vi "GetEventForceActuatorWarningField.vi"(10 "Event Data":string, 11 "Cluster in":refnum<vi>) -> (3 "Array":string[](array[string]))   [LabVIEW 2016]
uses:
  SALLV_m1m3/DataTypes/logevent_ForceActuatorWarning.ctl
  SALLV_m1m3/SALLV_m1m3.lvlib
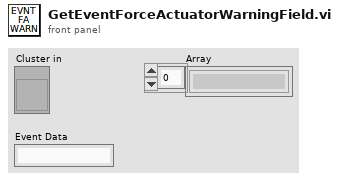
[diagram p1: front panel]
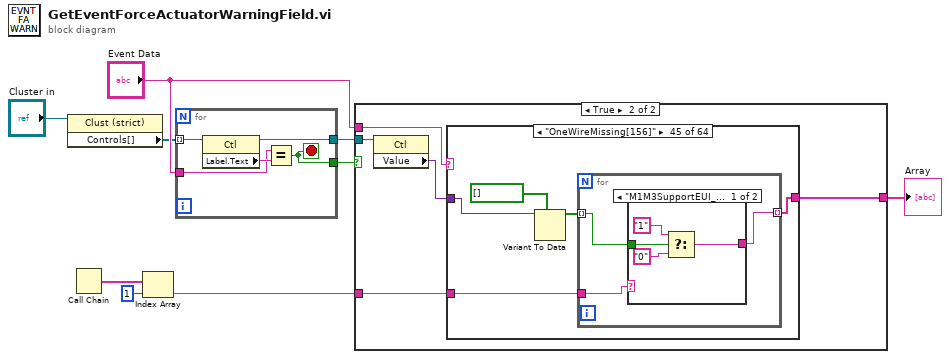
[diagram p0: block diagram]
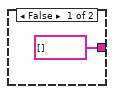
[diagram p2: hidden frame]
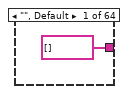
[diagram p3: hidden frame]
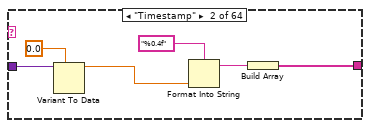
[diagram p4: hidden frame]
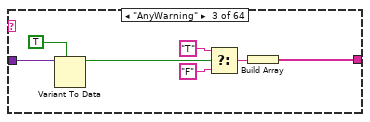
[diagram p5: hidden frame]
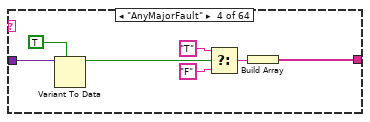
[diagram p6: hidden frame]
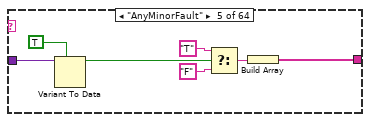
[diagram p7: hidden frame]
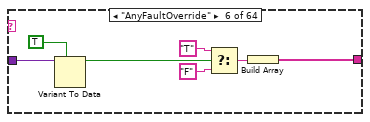
[diagram p8: hidden frame]
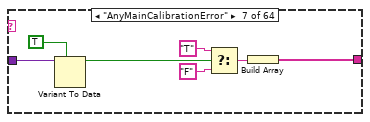
[diagram p9: hidden frame]
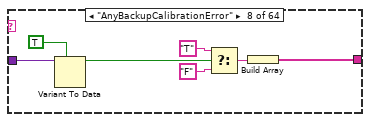
[diagram p10: hidden frame]
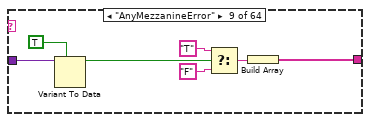
[diagram p11: hidden frame]
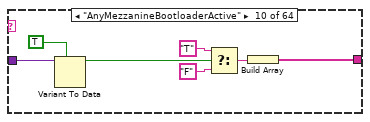
[diagram p12: hidden frame]
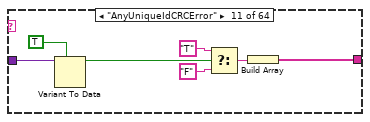
[diagram p13: hidden frame]
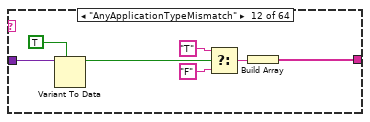
[diagram p14: hidden frame]
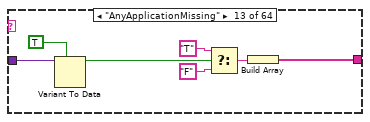
[diagram p15: hidden frame]
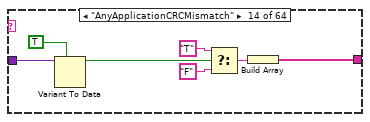
[diagram p16: hidden frame]
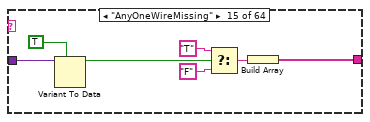
[diagram p17: hidden frame]
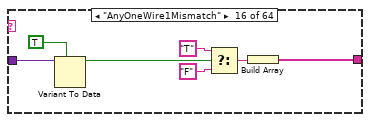
[diagram p18: hidden frame]
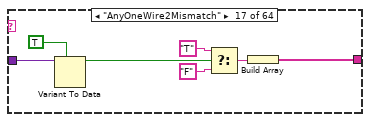
[diagram p19: hidden frame]
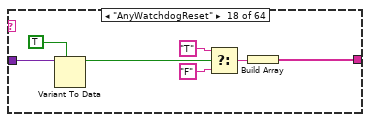
[diagram p20: hidden frame]
diagram:
  n1 = property on="Property Node" class="Clust (strict)"(reference="Cluster in") -> ("Controls[]"=w6:refnum<vi>[])  [unwired: 1 in, 2 out]
  n2 = Call Chain() -> (call chain=w2:string[])
  n3 = Index Array(array=w2, index=1) -> (element=w1:string)
  n4 = for {
    tunnel: w6 -> [w14] mode=indexing
    tunnel: [w13] -> w8
    tunnel: "Event Data" -> [w11]
    tunnel: [w10] -> w9
    stop <- w10 stop-if-true
    n5 = property on="Property Node" class="Ctl"(reference=w14) -> (reference out=w13:refnum<vi>, "Label.Text"=w12:string)  [unwired: 1 in, 1 out]
    n6 = Equal?(x=w11, y=w12) -> (x = y?=w10:bool)
  }
  n7 = case shown="True" w9 {
    tunnel: "Event Data" -> [_ w20]
    tunnel: w8 -> [_ w19]
    tunnel: [string[] [] w17] -> w5
    tunnel: w1 -> [_ w16]
    frame False {
    }
    frame True {
      n8 = property on="Property Node" class="Ctl"(reference=w19) -> ("Value"=w18:variant)  [unwired: 1 in, 2 out]
      n9 = case shown="\"OneWireMissing[156]\"" w20 {
        tunnel: [string[] [] w25 w28 w35 w42 w49 w56 w63 w70 w77 w84 w91 w98 w105 w112 w119 w126 w133 w140 w147 w154 w161 w168 w175 w182 w189 w196 w203 w210 w217 w224 w231 w238 w246 w262 w278 w294 w310 w326 w342 w358 w374 w390 w406 w422 w438 w454 w470 w486 w502 w518 w534 w550 w566 w582 w598 w614 w630 w646 w662 w678 w694 w710 w728] -> w17
        tunnel: w18 -> [_ w23 w34 w41 w48 w55 w62 w69 w76 w83 w90 w97 w104 w111 w118 w125 w132 w139 w146 w153 w160 w167 w174 w181 w188 w195 w202 w209 w216 w223 w230 w237 w244 w249 w265 w281 w297 w313 w329 w345 w361 w377 w393 w409 w425 w441 w457 w473 w489 w505 w521 w537 w553 w569 w585 w601 w617 w633 w649 w665 w681 w697 w713 w726]
        tunnel: w16 -> [_ _ _ _ _ _ _ _ _ _ _ _ _ _ _ _ _ _ _ _ _ _ _ _ _ _ _ _ _ _ _ _ _ w245 w261 w277 w293 w309 w325 w341 w357 w373 w389 w405 w421 w437 w453 w469 w485 w501 w517 w533 w549 w565 w581 w597 w613 w629 w645 w661 w677 w693 w709 _]
        frame "", Default {
        }
        frame "Timestamp" {
          n10 = Variant To Data(type=0.0, Variant=w23) -> (data=w24:dbl)  [unwired: 1 in, 1 out]
          n11 = Format Into String(format string="%0.4f", w24) -> (resulting string=w26:string)  [unwired: 2 in, 1 out]
          n12 = Build Array(w26) -> (w25:string[])
        }
        frame "AnyWarning" {
          n13 = Variant To Data(type=TRUE, Variant=w34) -> (data=w32:bool)  [unwired: 1 in, 1 out]
          n14 = Select(t="T", s=w32, f="F") -> (s? t:f=w29:string)
          n15 = Build Array(w29) -> (w28:string[])
        }
        frame "AnyMajorFault" {
          n16 = Variant To Data(type=TRUE, Variant=w41) -> (data=w39:bool)  [unwired: 1 in, 1 out]
          n17 = Select(t="T", s=w39, f="F") -> (s? t:f=w36:string)
          n18 = Build Array(w36) -> (w35:string[])
        }
        frame "AnyMinorFault" {
          n19 = Variant To Data(type=TRUE, Variant=w48) -> (data=w46:bool)  [unwired: 1 in, 1 out]
          n20 = Select(t="T", s=w46, f="F") -> (s? t:f=w43:string)
          n21 = Build Array(w43) -> (w42:string[])
        }
        frame "AnyFaultOverride" {
          n22 = Variant To Data(type=TRUE, Variant=w55) -> (data=w53:bool)  [unwired: 1 in, 1 out]
          n23 = Select(t="T", s=w53, f="F") -> (s? t:f=w50:string)
          n24 = Build Array(w50) -> (w49:string[])
        }
        frame "AnyMainCalibrationError" {
          n25 = Variant To Data(type=TRUE, Variant=w62) -> (data=w60:bool)  [unwired: 1 in, 1 out]
          n26 = Select(t="T", s=w60, f="F") -> (s? t:f=w57:string)
          n27 = Build Array(w57) -> (w56:string[])
        }
        frame "AnyBackupCalibrationError" {
          n28 = Variant To Data(type=TRUE, Variant=w69) -> (data=w67:bool)  [unwired: 1 in, 1 out]
          n29 = Select(t="T", s=w67, f="F") -> (s? t:f=w64:string)
          n30 = Build Array(w64) -> (w63:string[])
        }
        frame "AnyMezzanineError" {
          n31 = Variant To Data(type=TRUE, Variant=w76) -> (data=w74:bool)  [unwired: 1 in, 1 out]
          n32 = Select(t="T", s=w74, f="F") -> (s? t:f=w71:string)
          n33 = Build Array(w71) -> (w70:string[])
        }
        frame "AnyMezzanineBootloaderActive" {
          n34 = Variant To Data(type=TRUE, Variant=w83) -> (data=w81:bool)  [unwired: 1 in, 1 out]
          n35 = Select(t="T", s=w81, f="F") -> (s? t:f=w78:string)
          n36 = Build Array(w78) -> (w77:string[])
        }
        frame "AnyUniqueIdCRCError" {
          n37 = Variant To Data(type=TRUE, Variant=w90) -> (data=w88:bool)  [unwired: 1 in, 1 out]
          n38 = Select(t="T", s=w88, f="F") -> (s? t:f=w85:string)
          n39 = Build Array(w85) -> (w84:string[])
        }
        frame "AnyApplicationTypeMismatch" {
          n40 = Variant To Data(type=TRUE, Variant=w97) -> (data=w95:bool)  [unwired: 1 in, 1 out]
          n41 = Select(t="T", s=w95, f="F") -> (s? t:f=w92:string)
          n42 = Build Array(w92) -> (w91:string[])
        }
        frame "AnyApplicationMissing" {
          n43 = Variant To Data(type=TRUE, Variant=w104) -> (data=w102:bool)  [unwired: 1 in, 1 out]
          n44 = Select(t="T", s=w102, f="F") -> (s? t:f=w99:string)
          n45 = Build Array(w99) -> (w98:string[])
        }
        frame "AnyApplicationCRCMismatch" {
          n46 = Variant To Data(type=TRUE, Variant=w111) -> (data=w109:bool)  [unwired: 1 in, 1 out]
          n47 = Select(t="T", s=w109, f="F") -> (s? t:f=w106:string)
          n48 = Build Array(w106) -> (w105:string[])
        }
        frame "AnyOneWireMissing" {
          n49 = Variant To Data(type=TRUE, Variant=w118) -> (data=w116:bool)  [unwired: 1 in, 1 out]
          n50 = Select(t="T", s=w116, f="F") -> (s? t:f=w113:string)
          n51 = Build Array(w113) -> (w112:string[])
        }
        frame "AnyOneWire1Mismatch" {
          n52 = Variant To Data(type=TRUE, Variant=w125) -> (data=w123:bool)  [unwired: 1 in, 1 out]
          n53 = Select(t="T", s=w123, f="F") -> (s? t:f=w120:string)
          n54 = Build Array(w120) -> (w119:string[])
        }
        frame "AnyOneWire2Mismatch" {
          n55 = Variant To Data(type=TRUE, Variant=w132) -> (data=w130:bool)  [unwired: 1 in, 1 out]
          n56 = Select(t="T", s=w130, f="F") -> (s? t:f=w127:string)
          n57 = Build Array(w127) -> (w126:string[])
        }
        frame "AnyWatchdogReset" {
          n58 = Variant To Data(type=TRUE, Variant=w139) -> (data=w137:bool)  [unwired: 1 in, 1 out]
          n59 = Select(t="T", s=w137, f="F") -> (s? t:f=w134:string)
          n60 = Build Array(w134) -> (w133:string[])
        }
        frame "AnyBrownOut" {
          n61 = Variant To Data(type=TRUE, Variant=w146) -> (data=w144:bool)  [unwired: 1 in, 1 out]
          n62 = Select(t="T", s=w144, f="F") -> (s? t:f=w141:string)
          n63 = Build Array(w141) -> (w140:string[])
        }
        frame "AnyEventTrapReset" {
          n64 = Variant To Data(type=TRUE, Variant=w153) -> (data=w151:bool)  [unwired: 1 in, 1 out]
          n65 = Select(t="T", s=w151, f="F") -> (s? t:f=w148:string)
          n66 = Build Array(w148) -> (w147:string[])
        }
        frame "AnySSRPowerFault" {
          n67 = Variant To Data(type=TRUE, Variant=w160) -> (data=w158:bool)  [unwired: 1 in, 1 out]
          n68 = Select(t="T", s=w158, f="F") -> (s? t:f=w155:string)
          n69 = Build Array(w155) -> (w154:string[])
        }
        frame "AnyAuxPowerFault" {
          n70 = Variant To Data(type=TRUE, Variant=w167) -> (data=w165:bool)  [unwired: 1 in, 1 out]
          n71 = Select(t="T", s=w165, f="F") -> (s? t:f=w162:string)
          n72 = Build Array(w162) -> (w161:string[])
        }
        frame "AnyMezzaninePowerFault" {
          n73 = Variant To Data(type=TRUE, Variant=w174) -> (data=w172:bool)  [unwired: 1 in, 1 out]
          n74 = Select(t="T", s=w172, f="F") -> (s? t:f=w169:string)
          n75 = Build Array(w169) -> (w168:string[])
        }
        frame "AnyMezzanineCurrentAmp1Fault" {
          n76 = Variant To Data(type=TRUE, Variant=w181) -> (data=w179:bool)  [unwired: 1 in, 1 out]
          n77 = Select(t="T", s=w179, f="F") -> (s? t:f=w176:string)
          n78 = Build Array(w176) -> (w175:string[])
        }
        frame "AnyMezzanineCurrentAmp2Fault" {
          n79 = Variant To Data(type=TRUE, Variant=w188) -> (data=w186:bool)  [unwired: 1 in, 1 out]
          n80 = Select(t="T", s=w186, f="F") -> (s? t:f=w183:string)
          n81 = Build Array(w183) -> (w182:string[])
        }
        frame "AnyMezzanineUniqueIdCRCError" {
          n82 = Variant To Data(type=TRUE, Variant=w195) -> (data=w193:bool)  [unwired: 1 in, 1 out]
          n83 = Select(t="T", s=w193, f="F") -> (s? t:f=w190:string)
          n84 = Build Array(w190) -> (w189:string[])
        }
        frame "AnyMezzanineMainCalibrationError" {
          n85 = Variant To Data(type=TRUE, Variant=w202) -> (data=w200:bool)  [unwired: 1 in, 1 out]
          n86 = Select(t="T", s=w200, f="F") -> (s? t:f=w197:string)
          n87 = Build Array(w197) -> (w196:string[])
        }
        frame "AnyMezzanineBackupCalibrationError" {
          n88 = Variant To Data(type=TRUE, Variant=w209) -> (data=w207:bool)  [unwired: 1 in, 1 out]
          n89 = Select(t="T", s=w207, f="F") -> (s? t:f=w204:string)
          n90 = Build Array(w204) -> (w203:string[])
        }
        frame "AnyMezzanineEventTrapReset" {
          n91 = Variant To Data(type=TRUE, Variant=w216) -> (data=w214:bool)  [unwired: 1 in, 1 out]
          n92 = Select(t="T", s=w214, f="F") -> (s? t:f=w211:string)
          n93 = Build Array(w211) -> (w210:string[])
        }
        frame "AnyMezzanineApplicationMissing" {
          n94 = Variant To Data(type=TRUE, Variant=w223) -> (data=w221:bool)  [unwired: 1 in, 1 out]
          n95 = Select(t="T", s=w221, f="F") -> (s? t:f=w218:string)
          n96 = Build Array(w218) -> (w217:string[])
        }
        frame "AnyMezzanineApplicationCRCMismatch" {
          n97 = Variant To Data(type=TRUE, Variant=w230) -> (data=w228:bool)  [unwired: 1 in, 1 out]
          n98 = Select(t="T", s=w228, f="F") -> (s? t:f=w225:string)
          n99 = Build Array(w225) -> (w224:string[])
        }
        frame "AnyILCFault" {
          n100 = Variant To Data(type=TRUE, Variant=w237) -> (data=w235:bool)  [unwired: 1 in, 1 out]
          n101 = Select(t="T", s=w235, f="F") -> (s? t:f=w232:string)
          n102 = Build Array(w232) -> (w231:string[])
        }
        frame "AnyBroadcastCounterWarning" {
          n103 = Variant To Data(type=TRUE, Variant=w244) -> (data=w242:bool)  [unwired: 1 in, 1 out]
          n104 = Select(t="T", s=w242, f="F") -> (s? t:f=w239:string)
          n105 = Build Array(w239) -> (w238:string[])
        }
        frame "MajorFault[156]" {
          n106 = Variant To Data(type=bool[] [], Variant=w249) -> (data=w247:bool[])  [unwired: 1 in, 1 out]
          n107 = for {
            tunnel: w247 -> [w252] mode=indexing
            tunnel: [w251] -> w246 mode=indexing
            tunnel: w245 -> [w250]
            n108 = case shown="\"M1M3SupportEUI_Views.lvlib:FA Graphic View.vi\"" w250 {
              tunnel: w252 -> [w256 w260]
              tunnel: [w255 w257] -> w251
              frame "M1M3SupportEUI_Views.lvlib:FA Graphic View.vi" {
                n109 = Select(t="1", s=w256, f="0") -> (s? t:f=w255:string)
              }
              frame "", Default {
                n110 = Select(t="T", s=w260, f="F") -> (s? t:f=w257:string)
              }
            }
          }
        }
        frame "MinorFault[156]" {
          n111 = Variant To Data(type=bool[] [], Variant=w265) -> (data=w263:bool[])  [unwired: 1 in, 1 out]
          n112 = for {
            tunnel: w263 -> [w268] mode=indexing
            tunnel: [w267] -> w262 mode=indexing
            tunnel: w261 -> [w266]
            n113 = case shown="\"M1M3SupportEUI_Views.lvlib:FA Graphic View.vi\"" w266 {
              tunnel: w268 -> [w272 w276]
              tunnel: [w271 w273] -> w267
              frame "M1M3SupportEUI_Views.lvlib:FA Graphic View.vi" {
                n114 = Select(t="1", s=w272, f="0") -> (s? t:f=w271:string)
              }
              frame "", Default {
                n115 = Select(t="T", s=w276, f="F") -> (s? t:f=w273:string)
              }
            }
          }
        }
        frame "FaultOverride[156]" {
          n116 = Variant To Data(type=bool[] [], Variant=w281) -> (data=w279:bool[])  [unwired: 1 in, 1 out]
          n117 = for {
            tunnel: w279 -> [w284] mode=indexing
            tunnel: [w282] -> w278 mode=indexing
            tunnel: w277 -> [w283]
            n118 = case shown="\"M1M3SupportEUI_Views.lvlib:FA Graphic View.vi\"" w283 {
              tunnel: w284 -> [w288 w292]
              tunnel: [w287 w289] -> w282
              frame "M1M3SupportEUI_Views.lvlib:FA Graphic View.vi" {
                n119 = Select(t="1", s=w288, f="0") -> (s? t:f=w287:string)
              }
              frame Default {
                n120 = Select(t="T", s=w292, f="F") -> (s? t:f=w289:string)
              }
            }
          }
        }
        frame "MainCalibrationError[156]" {
          n121 = Variant To Data(type=bool[] [], Variant=w297) -> (data=w295:bool[])  [unwired: 1 in, 1 out]
          n122 = for {
            tunnel: w295 -> [w300] mode=indexing
            tunnel: [w299] -> w294 mode=indexing
            tunnel: w293 -> [w298]
            n123 = case shown="\"M1M3SupportEUI_Views.lvlib:FA Graphic View.vi\"" w298 {
              tunnel: w300 -> [w304 w308]
              tunnel: [w303 w305] -> w299
              frame "M1M3SupportEUI_Views.lvlib:FA Graphic View.vi" {
                n124 = Select(t="1", s=w304, f="0") -> (s? t:f=w303:string)
              }
              frame "", Default {
                n125 = Select(t="T", s=w308, f="F") -> (s? t:f=w305:string)
              }
            }
          }
        }
        frame "BackupCalibrationError[156]" {
          n126 = Variant To Data(type=bool[] [], Variant=w313) -> (data=w311:bool[])  [unwired: 1 in, 1 out]
          n127 = for {
            tunnel: w311 -> [w316] mode=indexing
            tunnel: [w314] -> w310 mode=indexing
            tunnel: w309 -> [w315]
            n128 = case shown="\"M1M3SupportEUI_Views.lvlib:FA Graphic View.vi\"" w315 {
              tunnel: w316 -> [w320 w324]
              tunnel: [w319 w321] -> w314
              frame "M1M3SupportEUI_Views.lvlib:FA Graphic View.vi" {
                n129 = Select(t="1", s=w320, f="0") -> (s? t:f=w319:string)
              }
              frame Default {
                n130 = Select(t="T", s=w324, f="F") -> (s? t:f=w321:string)
              }
            }
          }
        }
        frame "MezzanineError[156]" {
          n131 = Variant To Data(type=bool[] [], Variant=w329) -> (data=w327:bool[])  [unwired: 1 in, 1 out]
          n132 = for {
            tunnel: w327 -> [w332] mode=indexing
            tunnel: [w331] -> w326 mode=indexing
            tunnel: w325 -> [w330]
            n133 = case shown="\"M1M3SupportEUI_Views.lvlib:FA Graphic View.vi\"" w330 {
              tunnel: w332 -> [w336 w340]
              tunnel: [w335 w337] -> w331
              frame "M1M3SupportEUI_Views.lvlib:FA Graphic View.vi" {
                n134 = Select(t="1", s=w336, f="0") -> (s? t:f=w335:string)
              }
              frame "", Default {
                n135 = Select(t="T", s=w340, f="F") -> (s? t:f=w337:string)
              }
            }
          }
        }
        frame "MezzanineBootloaderActive[156]" {
          n136 = Variant To Data(type=bool[] [], Variant=w345) -> (data=w343:bool[])  [unwired: 1 in, 1 out]
          n137 = for {
            tunnel: w343 -> [w348] mode=indexing
            tunnel: [w347] -> w342 mode=indexing
            tunnel: w341 -> [w346]
            n138 = case shown="\"M1M3SupportEUI_Views.lvlib:FA Graphic View.vi\"" w346 {
              tunnel: w348 -> [w352 w356]
              tunnel: [w351 w353] -> w347
              frame "M1M3SupportEUI_Views.lvlib:FA Graphic View.vi" {
                n139 = Select(t="1", s=w352, f="0") -> (s? t:f=w351:string)
              }
              frame "", Default {
                n140 = Select(t="T", s=w356, f="F") -> (s? t:f=w353:string)
              }
            }
          }
        }
        frame "UniqueIdCRCError[156]" {
          n141 = Variant To Data(type=bool[] [], Variant=w361) -> (data=w359:bool[])  [unwired: 1 in, 1 out]
          n142 = for {
            tunnel: w359 -> [w364] mode=indexing
            tunnel: [w363] -> w358 mode=indexing
            tunnel: w357 -> [w362]
            n143 = case shown="\"M1M3SupportEUI_Views.lvlib:FA Graphic View.vi\"" w362 {
              tunnel: w364 -> [w368 w372]
              tunnel: [w367 w369] -> w363
              frame "M1M3SupportEUI_Views.lvlib:FA Graphic View.vi" {
                n144 = Select(t="1", s=w368, f="0") -> (s? t:f=w367:string)
              }
              frame "", Default {
                n145 = Select(t="T", s=w372, f="F") -> (s? t:f=w369:string)
              }
            }
          }
        }
        frame "ApplicationTypeMismatch[156]" {
          n146 = Variant To Data(type=bool[] [], Variant=w377) -> (data=w375:bool[])  [unwired: 1 in, 1 out]
          n147 = for {
            tunnel: w375 -> [w380] mode=indexing
            tunnel: [w379] -> w374 mode=indexing
            tunnel: w373 -> [w378]
            n148 = case shown="\"M1M3SupportEUI_Views.lvlib:FA Graphic View.vi\"" w378 {
              tunnel: w380 -> [w384 w388]
              tunnel: [w383 w385] -> w379
              frame "M1M3SupportEUI_Views.lvlib:FA Graphic View.vi" {
                n149 = Select(t="1", s=w384, f="0") -> (s? t:f=w383:string)
              }
              frame "", Default {
                n150 = Select(t="T", s=w388, f="F") -> (s? t:f=w385:string)
              }
            }
          }
        }
        frame "ApplicationMissing[156]" {
          n151 = Variant To Data(type=bool[] [], Variant=w393) -> (data=w391:bool[])  [unwired: 1 in, 1 out]
          n152 = for {
            tunnel: w391 -> [w396] mode=indexing
            tunnel: [w395] -> w390 mode=indexing
            tunnel: w389 -> [w394]
            n153 = case shown="\"M1M3SupportEUI_Views.lvlib:FA Graphic View.vi\"" w394 {
              tunnel: w396 -> [w400 w404]
              tunnel: [w399 w401] -> w395
              frame "M1M3SupportEUI_Views.lvlib:FA Graphic View.vi" {
                n154 = Select(t="1", s=w400, f="0") -> (s? t:f=w399:string)
              }
              frame "", Default {
                n155 = Select(t="T", s=w404, f="F") -> (s? t:f=w401:string)
              }
            }
          }
        }
        frame "ApplicationCRCMismatch[156]" {
          n156 = Variant To Data(type=bool[] [], Variant=w409) -> (data=w407:bool[])  [unwired: 1 in, 1 out]
          n157 = for {
            tunnel: w407 -> [w412] mode=indexing
            tunnel: [w410] -> w406 mode=indexing
            tunnel: w405 -> [w411]
            n158 = case shown="\"M1M3SupportEUI_Views.lvlib:FA Graphic View.vi\"" w411 {
              tunnel: w412 -> [w416 w420]
              tunnel: [w415 w417] -> w410
              frame "M1M3SupportEUI_Views.lvlib:FA Graphic View.vi" {
                n159 = Select(t="1", s=w416, f="0") -> (s? t:f=w415:string)
              }
              frame Default {
                n160 = Select(t="T", s=w420, f="F") -> (s? t:f=w417:string)
              }
            }
          }
        }
        frame "OneWireMissing[156]" {
          n161 = Variant To Data(type=bool[] [], Variant=w425) -> (data=w423:bool[])  [unwired: 1 in, 1 out]
          n162 = for {
            tunnel: w423 -> [w428] mode=indexing
            tunnel: [w427] -> w422 mode=indexing
            tunnel: w421 -> [w426]
            n163 = case shown="\"M1M3SupportEUI_Views.lvlib:FA Graphic View.vi\"" w426 {
              tunnel: w428 -> [w432 w436]
              tunnel: [w431 w433] -> w427
              frame "M1M3SupportEUI_Views.lvlib:FA Graphic View.vi" {
                n164 = Select(t="1", s=w432, f="0") -> (s? t:f=w431:string)
              }
              frame "", Default {
                n165 = Select(t="T", s=w436, f="F") -> (s? t:f=w433:string)
              }
            }
          }
        }
        frame "OneWire1Mismatch[156]" {
          n166 = Variant To Data(type=bool[] [], Variant=w441) -> (data=w439:bool[])  [unwired: 1 in, 1 out]
          n167 = for {
            tunnel: w439 -> [w444] mode=indexing
            tunnel: [w443] -> w438 mode=indexing
            tunnel: w437 -> [w442]
            n168 = case shown="\"M1M3SupportEUI_Views.lvlib:FA Graphic View.vi\"" w442 {
              tunnel: w444 -> [w448 w452]
              tunnel: [w447 w449] -> w443
              frame "M1M3SupportEUI_Views.lvlib:FA Graphic View.vi" {
                n169 = Select(t="1", s=w448, f="0") -> (s? t:f=w447:string)
              }
              frame "", Default {
                n170 = Select(t="T", s=w452, f="F") -> (s? t:f=w449:string)
              }
            }
          }
        }
        frame "OneWire2Mismatch[156]" {
          n171 = Variant To Data(type=bool[] [], Variant=w457) -> (data=w455:bool[])  [unwired: 1 in, 1 out]
          n172 = for {
            tunnel: w455 -> [w460] mode=indexing
            tunnel: [w459] -> w454 mode=indexing
            tunnel: w453 -> [w458]
            n173 = case shown="\"M1M3SupportEUI_Views.lvlib:FA Graphic View.vi\"" w458 {
              tunnel: w460 -> [w464 w468]
              tunnel: [w463 w465] -> w459
              frame "M1M3SupportEUI_Views.lvlib:FA Graphic View.vi" {
                n174 = Select(t="1", s=w464, f="0") -> (s? t:f=w463:string)
              }
              frame "", Default {
                n175 = Select(t="T", s=w468, f="F") -> (s? t:f=w465:string)
              }
            }
          }
        }
        frame "WatchdogReset[156]" {
          n176 = Variant To Data(type=bool[] [], Variant=w473) -> (data=w471:bool[])  [unwired: 1 in, 1 out]
          n177 = for {
            tunnel: w471 -> [w476] mode=indexing
            tunnel: [w475] -> w470 mode=indexing
            tunnel: w469 -> [w474]
            n178 = case shown="\"M1M3SupportEUI_Views.lvlib:FA Graphic View.vi\"" w474 {
              tunnel: w476 -> [w480 w484]
              tunnel: [w479 w481] -> w475
              frame "M1M3SupportEUI_Views.lvlib:FA Graphic View.vi" {
                n179 = Select(t="1", s=w480, f="0") -> (s? t:f=w479:string)
              }
              frame "", Default {
                n180 = Select(t="T", s=w484, f="F") -> (s? t:f=w481:string)
              }
            }
          }
        }
        frame "BrownOut[156]" {
          n181 = Variant To Data(type=bool[] [], Variant=w489) -> (data=w487:bool[])  [unwired: 1 in, 1 out]
          n182 = for {
            tunnel: w487 -> [w492] mode=indexing
            tunnel: [w491] -> w486 mode=indexing
            tunnel: w485 -> [w490]
            n183 = case shown="\"M1M3SupportEUI_Views.lvlib:FA Graphic View.vi\"" w490 {
              tunnel: w492 -> [w496 w500]
              tunnel: [w495 w497] -> w491
              frame "M1M3SupportEUI_Views.lvlib:FA Graphic View.vi" {
                n184 = Select(t="1", s=w496, f="0") -> (s? t:f=w495:string)
              }
              frame "", Default {
                n185 = Select(t="T", s=w500, f="F") -> (s? t:f=w497:string)
              }
            }
          }
        }
        frame "EventTrapReset[156]" {
          n186 = Variant To Data(type=bool[] [], Variant=w505) -> (data=w503:bool[])  [unwired: 1 in, 1 out]
          n187 = for {
            tunnel: w503 -> [w508] mode=indexing
            tunnel: [w507] -> w502 mode=indexing
            tunnel: w501 -> [w506]
            n188 = case shown="\"M1M3SupportEUI_Views.lvlib:FA Graphic View.vi\"" w506 {
              tunnel: w508 -> [w512 w516]
              tunnel: [w511 w513] -> w507
              frame "M1M3SupportEUI_Views.lvlib:FA Graphic View.vi" {
                n189 = Select(t="1", s=w512, f="0") -> (s? t:f=w511:string)
              }
              frame "", Default {
                n190 = Select(t="T", s=w516, f="F") -> (s? t:f=w513:string)
              }
            }
          }
        }
        frame "SSRPowerFault[156]" {
          n191 = Variant To Data(type=bool[] [], Variant=w521) -> (data=w519:bool[])  [unwired: 1 in, 1 out]
          n192 = for {
            tunnel: w519 -> [w524] mode=indexing
            tunnel: [w523] -> w518 mode=indexing
            tunnel: w517 -> [w522]
            n193 = case shown="\"M1M3SupportEUI_Views.lvlib:FA Graphic View.vi\"" w522 {
              tunnel: w524 -> [w528 w532]
              tunnel: [w527 w529] -> w523
              frame "M1M3SupportEUI_Views.lvlib:FA Graphic View.vi" {
                n194 = Select(t="1", s=w528, f="0") -> (s? t:f=w527:string)
              }
              frame "", Default {
                n195 = Select(t="T", s=w532, f="F") -> (s? t:f=w529:string)
              }
            }
          }
        }
        frame "AuxPowerFault[156]" {
          n196 = Variant To Data(type=bool[] [], Variant=w537) -> (data=w535:bool[])  [unwired: 1 in, 1 out]
          n197 = for {
            tunnel: w535 -> [w540] mode=indexing
            tunnel: [w539] -> w534 mode=indexing
            tunnel: w533 -> [w538]
            n198 = case shown="\"M1M3SupportEUI_Views.lvlib:FA Graphic View.vi\"" w538 {
              tunnel: w540 -> [w544 w548]
              tunnel: [w543 w545] -> w539
              frame "M1M3SupportEUI_Views.lvlib:FA Graphic View.vi" {
                n199 = Select(t="1", s=w544, f="0") -> (s? t:f=w543:string)
              }
              frame "", Default {
                n200 = Select(t="T", s=w548, f="F") -> (s? t:f=w545:string)
              }
            }
          }
        }
        frame "MezzaninePowerFault[156]" {
          n201 = Variant To Data(type=bool[] [], Variant=w553) -> (data=w551:bool[])  [unwired: 1 in, 1 out]
          n202 = for {
            tunnel: w551 -> [w556] mode=indexing
            tunnel: [w555] -> w550 mode=indexing
            tunnel: w549 -> [w554]
            n203 = case shown="\"M1M3SupportEUI_Views.lvlib:FA Graphic View.vi\"" w554 {
              tunnel: w556 -> [w560 w564]
              tunnel: [w559 w561] -> w555
              frame "M1M3SupportEUI_Views.lvlib:FA Graphic View.vi" {
                n204 = Select(t="1", s=w560, f="0") -> (s? t:f=w559:string)
              }
              frame "", Default {
                n205 = Select(t="T", s=w564, f="F") -> (s? t:f=w561:string)
              }
            }
          }
        }
        frame "MezzanineCurrentAmp1Fault[156]" {
          n206 = Variant To Data(type=bool[] [], Variant=w569) -> (data=w567:bool[])  [unwired: 1 in, 1 out]
          n207 = for {
            tunnel: w567 -> [w572] mode=indexing
            tunnel: [w571] -> w566 mode=indexing
            tunnel: w565 -> [w570]
            n208 = case shown="\"M1M3SupportEUI_Views.lvlib:FA Graphic View.vi\"" w570 {
              tunnel: w572 -> [w576 w580]
              tunnel: [w575 w577] -> w571
              frame "M1M3SupportEUI_Views.lvlib:FA Graphic View.vi" {
                n209 = Select(t="1", s=w576, f="0") -> (s? t:f=w575:string)
              }
              frame "", Default {
                n210 = Select(t="T", s=w580, f="F") -> (s? t:f=w577:string)
              }
            }
          }
        }
        frame "MezzanineCurrentAmp2Fault[156]" {
          n211 = Variant To Data(type=bool[] [], Variant=w585) -> (data=w583:bool[])  [unwired: 1 in, 1 out]
          n212 = for {
            tunnel: w583 -> [w588] mode=indexing
            tunnel: [w587] -> w582 mode=indexing
            tunnel: w581 -> [w586]
            n213 = case shown="\"M1M3SupportEUI_Views.lvlib:FA Graphic View.vi\"" w586 {
              tunnel: w588 -> [w592 w596]
              tunnel: [w591 w593] -> w587
              frame "M1M3SupportEUI_Views.lvlib:FA Graphic View.vi" {
                n214 = Select(t="1", s=w592, f="0") -> (s? t:f=w591:string)
              }
              frame "", Default {
                n215 = Select(t="T", s=w596, f="F") -> (s? t:f=w593:string)
              }
            }
          }
        }
        frame "MezzanineUniqueIdCRCError[156]" {
          n216 = Variant To Data(type=bool[] [], Variant=w601) -> (data=w599:bool[])  [unwired: 1 in, 1 out]
          n217 = for {
            tunnel: w599 -> [w604] mode=indexing
            tunnel: [w603] -> w598 mode=indexing
            tunnel: w597 -> [w602]
            n218 = case shown="\"M1M3SupportEUI_Views.lvlib:FA Graphic View.vi\"" w602 {
              tunnel: w604 -> [w608 w612]
              tunnel: [w607 w609] -> w603
              frame "M1M3SupportEUI_Views.lvlib:FA Graphic View.vi" {
                n219 = Select(t="1", s=w608, f="0") -> (s? t:f=w607:string)
              }
              frame "", Default {
                n220 = Select(t="T", s=w612, f="F") -> (s? t:f=w609:string)
              }
            }
          }
        }
        frame "MezzanineMainCalibrationError[156]" {
          n221 = Variant To Data(type=bool[] [], Variant=w617) -> (data=w615:bool[])  [unwired: 1 in, 1 out]
          n222 = for {
            tunnel: w615 -> [w620] mode=indexing
            tunnel: [w619] -> w614 mode=indexing
            tunnel: w613 -> [w618]
            n223 = case shown="\"M1M3SupportEUI_Views.lvlib:FA Graphic View.vi\"" w618 {
              tunnel: w620 -> [w624 w628]
              tunnel: [w623 w625] -> w619
              frame "M1M3SupportEUI_Views.lvlib:FA Graphic View.vi" {
                n224 = Select(t="1", s=w624, f="0") -> (s? t:f=w623:string)
              }
              frame "", Default {
                n225 = Select(t="T", s=w628, f="F") -> (s? t:f=w625:string)
              }
            }
          }
        }
        frame "MezzanineBackupCalibrationError[156]" {
          n226 = Variant To Data(type=bool[] [], Variant=w633) -> (data=w631:bool[])  [unwired: 1 in, 1 out]
          n227 = for {
            tunnel: w631 -> [w636] mode=indexing
            tunnel: [w635] -> w630 mode=indexing
            tunnel: w629 -> [w634]
            n228 = case shown="\"M1M3SupportEUI_Views.lvlib:FA Graphic View.vi\"" w634 {
              tunnel: w636 -> [w640 w644]
              tunnel: [w639 w641] -> w635
              frame "M1M3SupportEUI_Views.lvlib:FA Graphic View.vi" {
                n229 = Select(t="1", s=w640, f="0") -> (s? t:f=w639:string)
              }
              frame "", Default {
                n230 = Select(t="T", s=w644, f="F") -> (s? t:f=w641:string)
              }
            }
          }
        }
        frame "MezzanineEventTrapReset[156]" {
          n231 = Variant To Data(type=bool[] [], Variant=w649) -> (data=w647:bool[])  [unwired: 1 in, 1 out]
          n232 = for {
            tunnel: w647 -> [w652] mode=indexing
            tunnel: [w651] -> w646 mode=indexing
            tunnel: w645 -> [w650]
            n233 = case shown="\"M1M3SupportEUI_Views.lvlib:FA Graphic View.vi\"" w650 {
              tunnel: w652 -> [w656 w660]
              tunnel: [w655 w657] -> w651
              frame "M1M3SupportEUI_Views.lvlib:FA Graphic View.vi" {
                n234 = Select(t="1", s=w656, f="0") -> (s? t:f=w655:string)
              }
              frame "", Default {
                n235 = Select(t="T", s=w660, f="F") -> (s? t:f=w657:string)
              }
            }
          }
        }
        frame "MezzanineApplicationMissing[156]" {
          n236 = Variant To Data(type=bool[] [], Variant=w665) -> (data=w663:bool[])  [unwired: 1 in, 1 out]
          n237 = for {
            tunnel: w663 -> [w668] mode=indexing
            tunnel: [w667] -> w662 mode=indexing
            tunnel: w661 -> [w666]
            n238 = case shown="\"M1M3SupportEUI_Views.lvlib:FA Graphic View.vi\"" w666 {
              tunnel: w668 -> [w672 w676]
              tunnel: [w671 w673] -> w667
              frame "M1M3SupportEUI_Views.lvlib:FA Graphic View.vi" {
                n239 = Select(t="1", s=w672, f="0") -> (s? t:f=w671:string)
              }
              frame "", Default {
                n240 = Select(t="T", s=w676, f="F") -> (s? t:f=w673:string)
              }
            }
          }
        }
        frame "MezzanineApplicationCRCMismatch[156]" {
          n241 = Variant To Data(type=bool[] [], Variant=w681) -> (data=w679:bool[])  [unwired: 1 in, 1 out]
          n242 = for {
            tunnel: w679 -> [w684] mode=indexing
            tunnel: [w682] -> w678 mode=indexing
            tunnel: w677 -> [w683]
            n243 = case shown="\"M1M3SupportEUI_Views.lvlib:FA Graphic View.vi\"" w683 {
              tunnel: w684 -> [w688 w692]
              tunnel: [w687 w689] -> w682
              frame "M1M3SupportEUI_Views.lvlib:FA Graphic View.vi" {
                n244 = Select(t="1", s=w688, f="0") -> (s? t:f=w687:string)
              }
              frame Default {
                n245 = Select(t="T", s=w692, f="F") -> (s? t:f=w689:string)
              }
            }
          }
        }
        frame "ILCFault[156]" {
          n246 = Variant To Data(type=bool[] [], Variant=w697) -> (data=w695:bool[])  [unwired: 1 in, 1 out]
          n247 = for {
            tunnel: w695 -> [w700] mode=indexing
            tunnel: [w699] -> w694 mode=indexing
            tunnel: w693 -> [w698]
            n248 = case shown="\"M1M3SupportEUI_Views.lvlib:FA Graphic View.vi\"" w698 {
              tunnel: w700 -> [w704 w708]
              tunnel: [w703 w705] -> w699
              frame "M1M3SupportEUI_Views.lvlib:FA Graphic View.vi" {
                n249 = Select(t="1", s=w704, f="0") -> (s? t:f=w703:string)
              }
              frame "", Default {
                n250 = Select(t="T", s=w708, f="F") -> (s? t:f=w705:string)
              }
            }
          }
        }
        frame "BroadcastCounterWarning[156]" {
          n251 = Variant To Data(type=bool[] [], Variant=w713) -> (data=w711:bool[])  [unwired: 1 in, 1 out]
          n252 = for {
            tunnel: w711 -> [w716] mode=indexing
            tunnel: [w715] -> w710 mode=indexing
            tunnel: w709 -> [w714]
            n253 = case shown="\"M1M3SupportEUI_Views.lvlib:FA Graphic View.vi\"" w714 {
              tunnel: w716 -> [w720 w724]
              tunnel: [w719 w721] -> w715
              frame "M1M3SupportEUI_Views.lvlib:FA Graphic View.vi" {
                n254 = Select(t="1", s=w720, f="0") -> (s? t:f=w719:string)
              }
              frame "", Default {
                n255 = Select(t="T", s=w724, f="F") -> (s? t:f=w721:string)
              }
            }
          }
        }
        frame "priority" {
          n256 = Variant To Data(type=0, Variant=w726) -> (data=w727:i32)  [unwired: 1 in, 1 out]
          n257 = Format Into String(format string="%d", w727) -> (resulting string=w729:string)  [unwired: 2 in, 1 out]
          n258 = Build Array(w729) -> (w728:string[])
        }
      }
    }
  }
  "Array" <- w5
